vi "Windowed Data1.vi"(11 "WaveformGraph in":refnum<vi>) -> (3 "Windowed num. of samples 2":dbl)   [LabVIEW 2014, in "Aquisicao de Dados.lvlib"]
uses:
  Aquisicao de Dados.lvlib
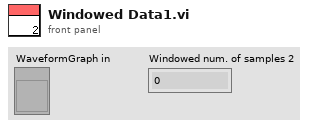
[diagram p1: front panel]
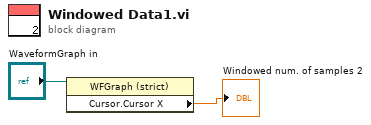
[diagram p0: block diagram]
diagram:
  n1 = property on="Property Node" class="WFGraph (strict)"(reference="WaveformGraph in") -> ("Cursor.Cursor X"=→"Windowed num. of samples 2":dbl)  [unwired: 1 in, 2 out]
